vi "Ini key read (Boolean).vi"(7 "Section":string, 8 "error in (no error)":errorcluster, 10 "Parameter names & setup":T2, 11 "Ini file refnum in":T1) -> (0 "error out":errorcluster, 2 "Value read/used":bool[](array[boolean]), 3 "Ini file refnum out":T1)   [LabVIEW 2020]
uses:
  Typedefs/Ini file interface (Boolean).ctl
  <vilib>/Utility/config.llb/Config Data RefNum.ctl
  <vilib>/Utility/config.llb/Read Key (Boolean).vi
  <vilib>/Utility/config.llb/Write Key (Boolean).vi
  <vilib>/Utility/config.llb/NI_LVConfig.lvlib
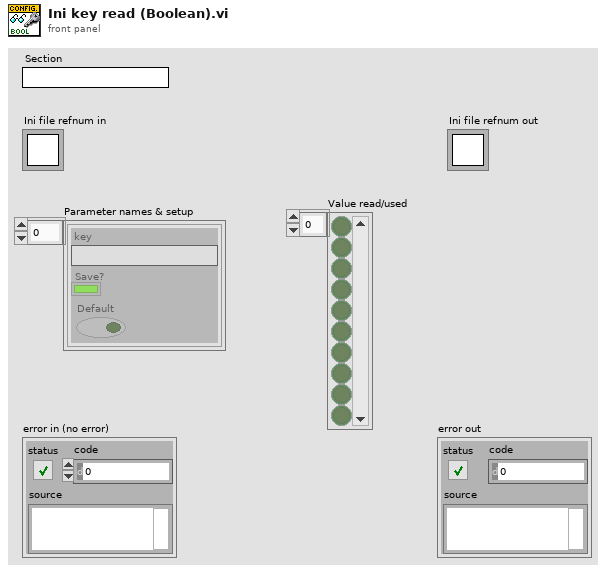
[diagram p1: front panel]
types:
  T1 = typedef "NI_LVConfig.lvlib/Config Data RefNum.ctl" = refnum<k1>
  T2 = typedef "Ini file interface (Boolean).ctl" = cluster{"key":string, "Save?":bool, "Default":bool}[]
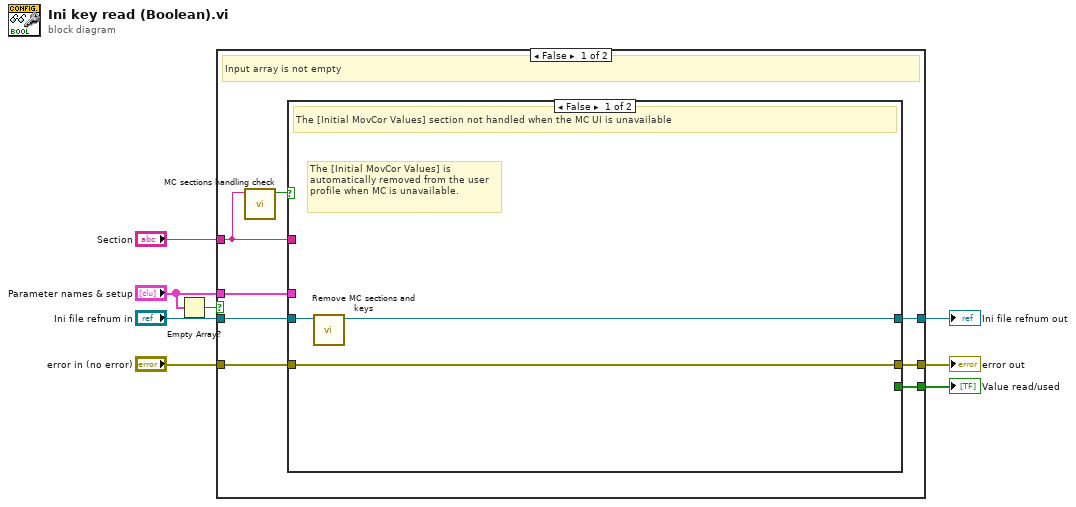
[diagram p0: block diagram]
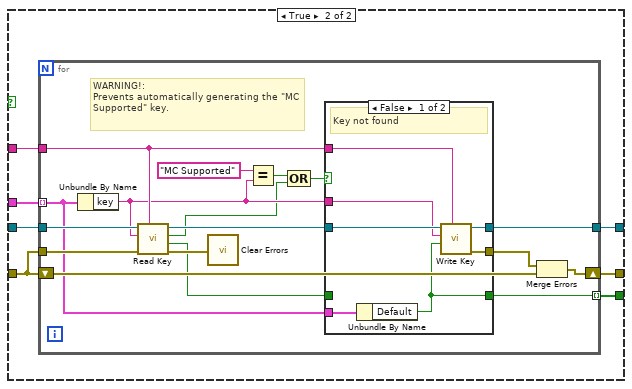
[diagram p2: hidden frame]
diagram:
  n1 = Empty Array?(array="Parameter names & setup") -> (empty?=w1:bool)
  n2 = case shown="False" w1 {
    tunnel: "Section" -> [w10 _]
    tunnel: "Parameter names & setup" -> [w16 _]
    tunnel: [w15 _] -> w7
    tunnel: "error in (no error)" -> [w14 w53]
    tunnel: [w13 w53] -> w5
    tunnel: [w12 w54] -> w4
    tunnel: "Ini file refnum in" -> [w11 w54]
    frame False {
      # "Input array is not empty"
      n3 = call "MC sections handling check.vi"("Section name"=w10) -> ("Section is \"Initial MovCor Values\" AND MC is supported"=w9:bool)  [unwired: 10 in]
      n4 = case shown="False" w9 {
        tunnel: w16 -> [_ w26]
        tunnel: [_ w25] -> w15
        tunnel: w14 -> [w19 w24]
        tunnel: [w19 w23] -> w13
        tunnel: [w17 w22] -> w12
        tunnel: w11 -> [w18 w21]
        tunnel: w10 -> [_ w20]
        frame False {
          # "The [Initial MovCor Values] is automatically removed from the user profile when MC is unavailable."
          # "The [Initial MovCor Values] section not handled when the MC UI is unavailable"
          n5 = call "Remove MC sections and keys.vi"("User profile ref"=w18) -> ("User profile ref"=w17:T1)  [unwired: 10 in]
        }
        frame True {
          n6 = for {
            tunnel: w20 -> [w32]
            tunnel: w21 -> [w43]
            tunnel: w24 -> [w42]
            tunnel: [w37] -> w22
            shift-right: [w41] -> w23
            shift-left: w24 -> [w40]
            tunnel: w26 -> [w33] mode=indexing
            tunnel: [w34] -> w25 mode=indexing
            # "WARNING!:\nPrevents automatically generating the \"MC Supported\" key."
            n7 = Unbundle By Name(w33) -> ("key"=w31:string)
            n8 = call-poly <vilib>:"Read Key.vi"("section"=w32, "error in (no error)"=w42, "key"=w31, "refnum"=w43) -> ("error out"=w39:errorcluster, "value"=w35:bool, "found?"=w28:bool, "refnum out"=w38:T1)  [unwired: 4 in]
            n9 = call <vilib>:"Clear Errors.vi"("error in (no error)"=w39) -> ()  [unwired: 5 in, 2 out]
            n10 = Equal?(x="MC Supported", y=w31) -> (x = y?=w29:bool)
            n11 = Compound Arithmetic op=OR(w29, w28) -> (w27:bool)
            n12 = case shown="False" w27 {
              tunnel: w38 -> [w50 w52]
              tunnel: [w49 w52] -> w37
              tunnel: [w48 _] -> w36
              tunnel: w32 -> [w47 _]
              tunnel: w31 -> [w46 _]
              tunnel: w35 -> [_ w51]
              tunnel: [w44 w51] -> w34
              tunnel: w33 -> [w45 _]
              frame False {
                # "Key not found"
                n13 = Unbundle By Name(w45) -> ("Default"=w44:bool)
                n14 = call-poly <vilib>:"Write Key.vi"("section"=w47, "value"=w44, "key"=w46, "refnum"=w50) -> ("error out"=w48:errorcluster, "refnum out"=w49:T1)  [unwired: 5 in, 1 out]
              }
              frame True {
                # "Key found or MC key"
              }
            }
            n15 = Merge Errors(w36, w40) -> (w41:errorcluster)
          }
        }
      }
    }
    frame True {
      # "Input array is empty"
    }
  }
  "Value read/used" <- w7
  "error out" <- w5
  "Ini file refnum out" <- w4
